vi "LP Filter.vi"(6 "Data rate":dbl, 9 "Time constant":dbl, 10 "New data":dbl, 11 "Previous data":dbl) -> (3 "Filtered data":dbl)   [LabVIEW 2021]
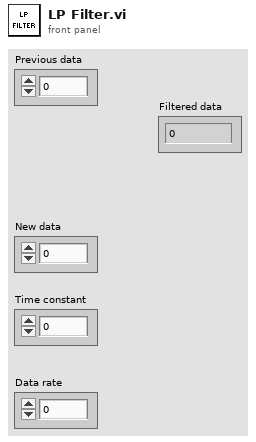
[diagram p1: front panel]
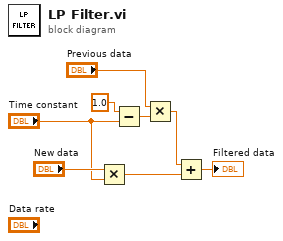
[diagram p0: block diagram]
diagram:
  n1 = Multiply(x="New data", y="Time constant") -> (x*y=w3:dbl)
  n2 = Subtract(x=1.0, y="Time constant") -> (x-y=w5:dbl)
  n3 = Multiply(x="Previous data", y=w5) -> (x*y=w4:dbl)
  n4 = Add(x=w4, y=w3) -> (x+y=→"Filtered data":dbl)
